vi "PanelParser.vi"(2 "VI reference":refnum<vi>) -> (7 "TreeItems[]":T2(array[cluster]), 9 "Ctrl":T1)   [LabVIEW 2021, in "Tree.lvlib" / "Tree.lvclass"]
uses:
  Tree.lvclass
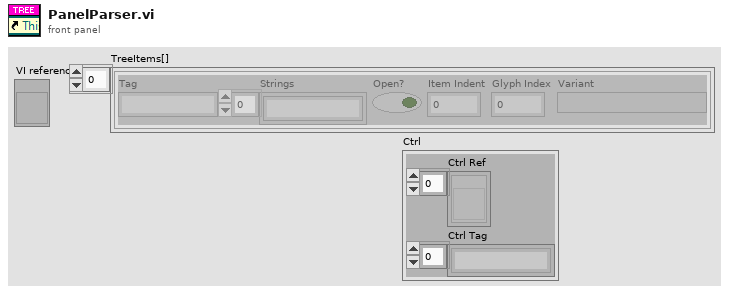
[diagram p1: front panel]
types:
  T1 = cluster{"Ctrl Ref":refnum<vi>[], "Ctrl Tag":string[]}
  T2 = cluster{"Tag":string, "Strings":string[], "Open?":bool, "Item Indent":i32, "Glyph Index":i32, "Variant":variant}[]
  T3 = cluster{"Left Cell String":string, "Child Text":string[], "Child Tag":string, "Item Indent":i32, "Child Only?":bool, "Glyph Index":i32}[]
  T4 = cluster{"Tag":string, "Strings":string[], "Open?":bool, "Item Indent":i32, "Glyph Index":i32, "Variant":variant}
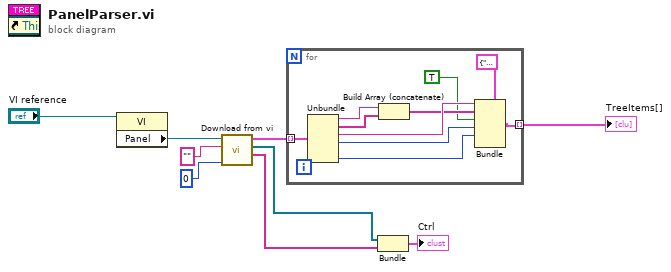
[diagram p0: block diagram]
diagram:
  n1 = property class="VI"(reference="VI reference") -> ("Panel"=w6:refnum<vi>)  [unwired: 1 in, 2 out]
  n2 = call "Download from vi.vi"("Indent Level"=0, "Parent tag"="", "Gen Refnum"=w6) -> ("Ctrl Tag"=w2:string[], "Ctrl Ref"=w3:refnum<vi>[], "appended array"=w9:T3)  [unwired: 6 in]
  n3 = for {
    tunnel: w9 -> [w19] mode=indexing
    tunnel: [w10] -> w4 mode=indexing
    n4 = Unbundle(w19) -> ("Left Cell String"=w16:string, "Child Text"=w15:string[], "Child Tag"=w17:string, "Item Indent"=w13:i32, "Glyph Index"=w12:i32)  [unwired: 1 out]
    n5 = Build Array (concatenate)(w16, w15) -> (w14:string[])
    n6 = Bundle(cluster=T4 {"Tag"="", "Strings"=[], "Open?"=FALSE, "Item Indent"=0, "Glyph Index"=0, "Variant"=variant} ("TreeItems[]"), "Tag"=w17, "Strings"=w14, "Open?"=TRUE, "Item Indent"=w13, "Glyph Index"=w12) -> (w10:T4)  [unwired: 1 in]
  }
  "TreeItems[]" <- w4
  n7 = Bundle("Ctrl Ref"=w3, "Ctrl Tag"=w2) -> (→"Ctrl":T1)  [unwired: 1 in]
